vi "File.Move File, Overwrite if Exists.vi"(8 "error in":errorcluster, 10 "Target Path":path, 11 "Source Path":path) -> (0 "error out":errorcluster, 3 "Target Out":path)   [LabVIEW 2018]
uses:
  Errors/Error.Error Code List.ctl
  <vilib>/KATE/Files/File Utils.lvlib
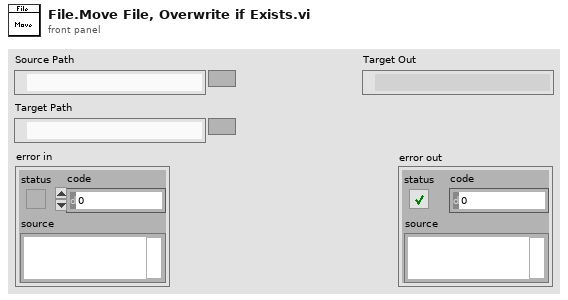
[diagram p1: front panel]
types:
  T1 = typedef "Error.Error Code List.ctl" = i32
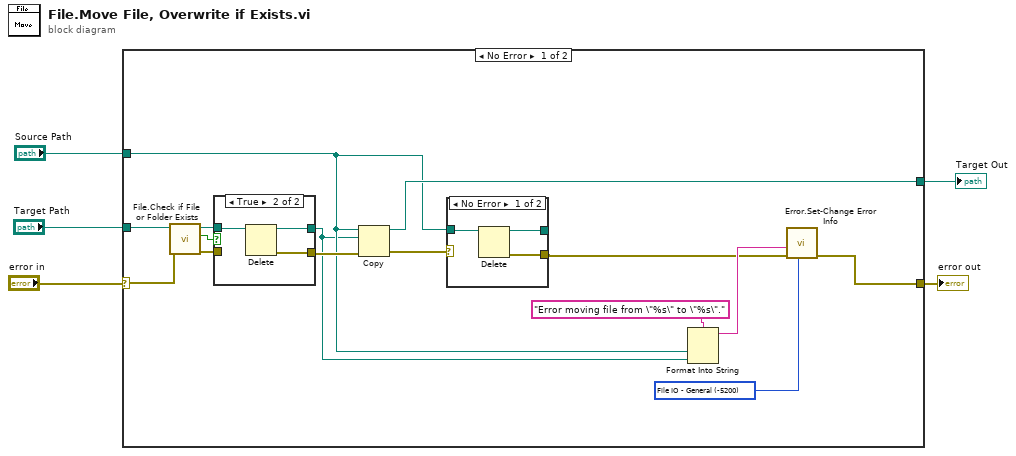
[diagram p0: block diagram]
diagram:
  n1 = case shown="No Error" "error in" {
    selector: "error in" -> [w16 w31]
    tunnel: "Target Path" -> [w18 w30]
    tunnel: [w6 w31] -> w4
    tunnel: "Source Path" -> [w9 _]
    tunnel: [w14 w30] -> w1
    frame No Error {
      w7 = T1 -5200 items=["No Error"=0, "Abort"=-2, "Misc"=-5000, "Fixture Error"=-5100, "File IO - General"=-5200, "FIle IO - Config Error"=-5201, "Instrument - General"=-5300, "Instrument - Serial Com"=-5301, "Instrument - Camera"=-5302, "Instrument - PS"=-5303, "Instrument - Oscilloscope"=-5304, "Instrument - Function Gen"=-5305, "Instrument - Load"=-5306, "Instrument - Meter"=-5307, "Instrument - Power Control"=-5308, "Instrument - Motion"=-5309, "Instrument - RF"=-5310, "System Exe"=-5400, "Image Processing"=-5500, "Communication"=-5600, "Script - Syntax Error"=-6000, "Script - Invalid Name or Param"=-6100, "Script - Timeout"=-6200, "Invalid Data"=-6300, "FW Update Error"=-6500] ("Std Code")
      n2 = call <vilib>:"File.Check if File or Folder Exists.vi"("error in"=w16, "Path"=w18) -> ("error out"=w17:errorcluster, "Exists"=w20:bool, "Dup Path"=w19:path)  [unwired: 5 in, 2 out]
      n3 = case shown="True" w20 {
        tunnel: w19 -> [w26 w29]
        tunnel: [_ w28] -> w15
        tunnel: [w26 w27] -> w8
        tunnel: w17 -> [_ _]
        frame False {
        }
        frame True {
          n4 = Delete(path (use dialog)=w29) -> (deleted path=w27:path, error out=w28:errorcluster)  [unwired: 4 in, 1 out]
        }
      }
      n5 = Copy(8:w15, 10:w8, 11:w9) -> (0:w13:errorcluster, 3:w14:path)  [unwired: 2 in, 1 out]
      n6 = case shown="No Error" w13 {
        selector: w13 -> [_ w24]
        tunnel: w9 -> [w23 w25]
        tunnel: [w22 w24] -> w10
        tunnel: [w21 w25] -> _
        frame No Error {
          n7 = Delete(path (use dialog)=w23) -> (deleted path=w21:path, error out=w22:errorcluster)  [unwired: 4 in, 1 out]
        }
        frame Error {
        }
      }
      n8 = Format Into String(format string="Error moving file from \"%s\" to \"%s\".", w9, w8) -> (resulting string=w11:string)  [unwired: 2 in, 1 out]
      n9 = call "Error.Set-Change Error Info.vi"("Std Code"=w7, "error in"=w10, "Description"=w11) -> ("error out"=w6:errorcluster)  [unwired: 8 in]
    }
    frame Error {
    }
  }
  "error out" <- w4
  "Target Out" <- w1
